vi "HAPS_PhaseSweep_Preamp.vi"() -> ()   [LabVIEW 2023, in "HAPS.lvlib"]
uses:
  HAPS.lvlib
  MCU_Function.ctl
  set_ele.ctl
  HAPS_SerialPort.ctl
  HAPS_MCU_ELE_Func.ctl
  R_S/R_S.lvlib
panel:
  in  "comn_gain":i32=17
  in  "ele_gain":i32=35
  in  "File_note":string
  in  "Init?":bool=TRUE
  out "Duration":dbl
  out "In-Phase : Phase(degree)":dbl[](graph)
  out "In-Phase : Gain(dB)":dbl[](graph)
  out "channel":i32
  out "chain_id":i32
  out "group":i32
  out "array_id":i32
  in  "Phase diff. Criteria":dbl format="%#_13g"
  in  "Tx/Rx":enum16{"Rx", "Tx"}(ring)=enum."Tx"
  in  "array_id (MCU index)":i32
  in  "MCU_UART_addr":refnum<visa-resource-name>="COM8"
  in  "Target(degree)":dbl format="%#_13g"
  in  "SweepPoints":i32=11
  in  "sParameter":i32=21
  in  "Stop_Freq(GHz)":dbl=39.5
  in  "Start_Freq(GHz)":dbl=38.5
  in  "VISA resource name":refnum<visa-resource-name>="TCPIP0::192.168.119.45::inst0::INSTR"
  in  "HAPS_Equipment":enum16{"Keysight", "R&S"}(ring)=enum."R&S"
  # "HAPS_24x24_Phase_Sweep_Preamp"
  # "VNA"
  # "Tx:35\nRx:22"
  # "DUT"
  # "4718.54"
  # "TCPIP0::192.168.1.31::hislip0::INSTR"
  # "Test Status"
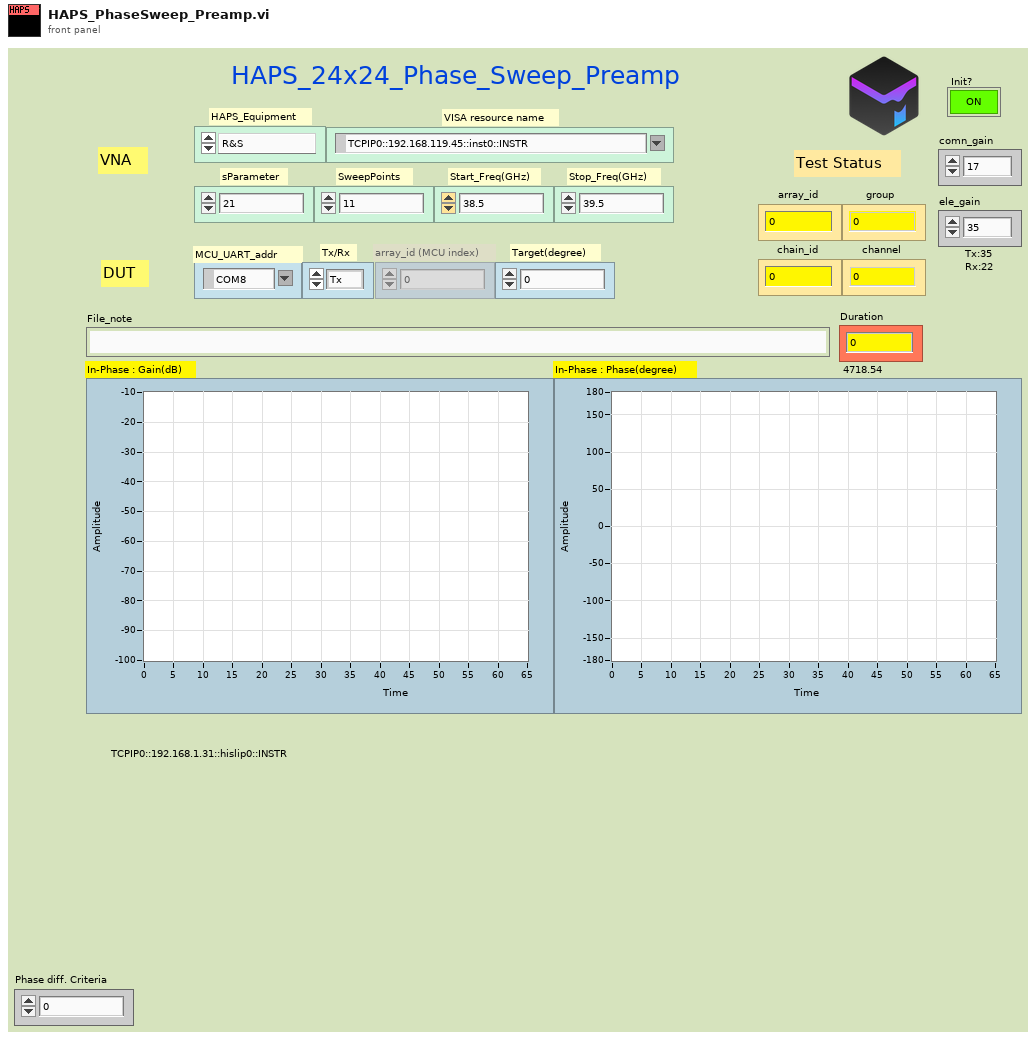
[diagram p1: front panel]
types:
  T1 = typedef "HAPS.lvlib/HAPS_SerialPort.ctl" = enum16{"Init", "Close", "CMD", "Flush"}
  T2 = typedef "HAPS.lvlib/HAPS_MCU_ELE_Func.ctl" = enum16{"array_init", "set_com_gain", "set_ch_gain_phase", "set_pd_range", "get_preamp_temp", "get_bfic_temp", "get_tx_pd", "ch_on", "ch_on_2", "ch_ctrl_all", "array_ctrl_src"}
  T3 = typedef "HAPS.lvlib/MCU_Function.ctl" = cluster{"Tx/Rx":enum16{"Rx", "Tx"}, "Enable?":enum16{"OFF", "On"}, "Source":enum16{"MCU", "ACU"}}
  T4 = typedef "HAPS.lvlib/set_ele.ctl" = cluster{"ch":i32, "chain_id":i32, "group":i32, "array_id":i32, "ele_phase":i32, "ele_gain":i32, "com_gain":i32, "pd_range":i32}
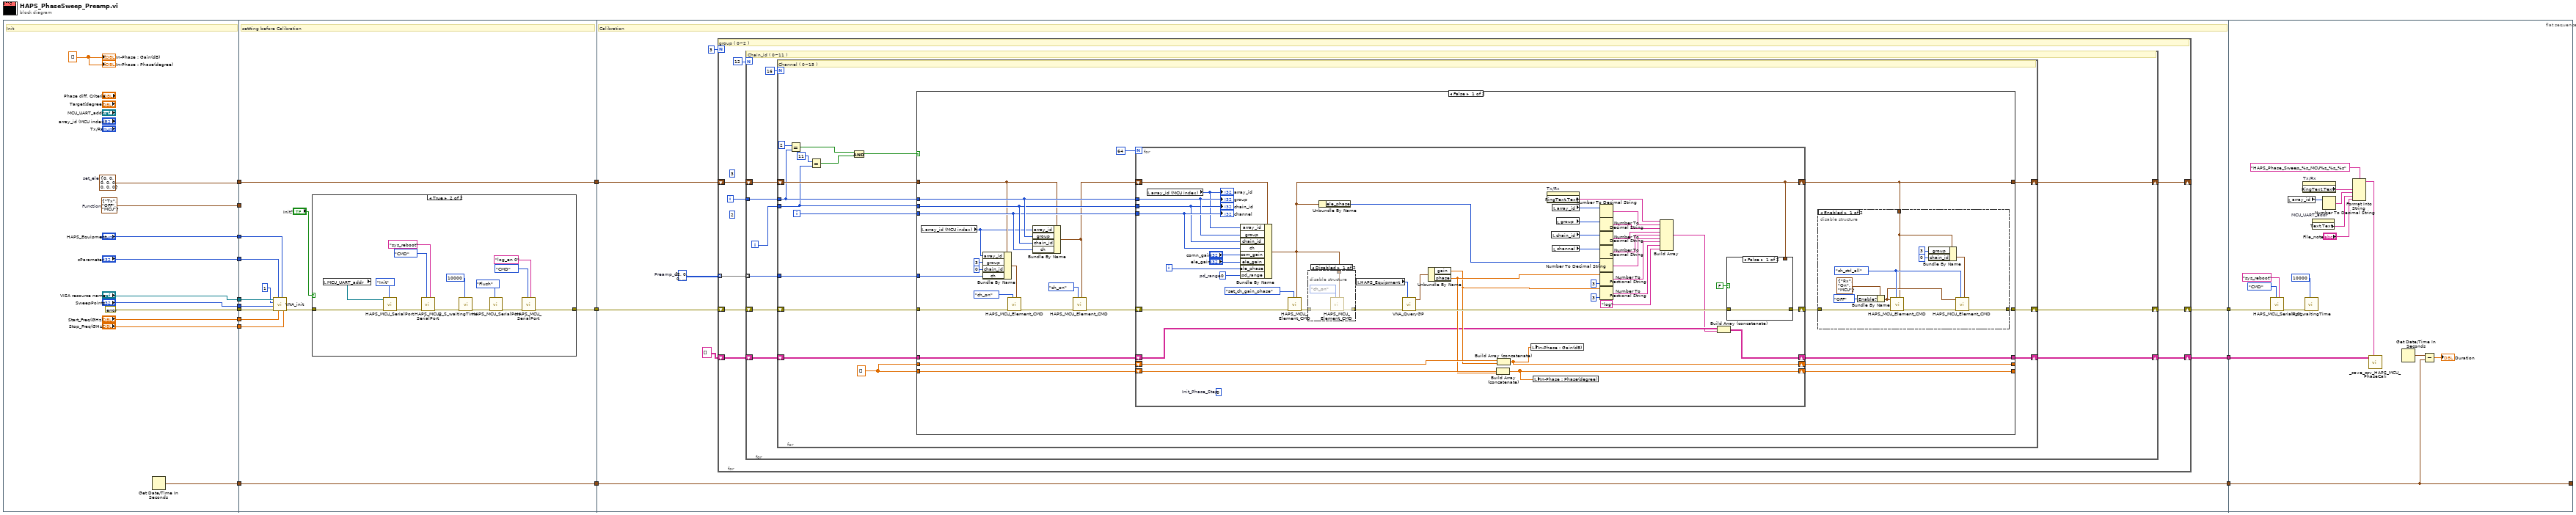
[diagram p0: block diagram]
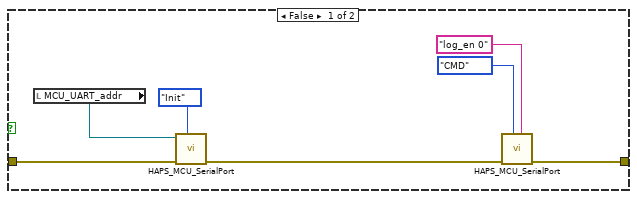
[diagram p2: hidden frame]
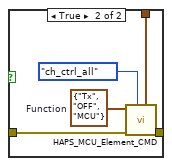
[diagram p5: hidden frame]
diagram:
  n1 = flat-sequence {
    tunnel: [w20] -> w16
    tunnel: [w27] -> w15
    tunnel: [errorcluster {"status"=FALSE, "code"=0, "source"=""} ("error in")] -> w13
    tunnel: ["sParameter"] -> w11
    tunnel: ["VISA resource name"] -> w10
    tunnel: ["Start_Freq(GHz)"] -> w9
    tunnel: ["Stop_Freq(GHz)"] -> w8
    tunnel: ["SweepPoints"] -> w7
    tunnel: ["HAPS_Equipment"] -> w6
    tunnel: [w17] -> w4
    tunnel: w16 -> [w40]
    tunnel: w15 -> [_]
    tunnel: [w40] -> w14
    tunnel: w13 -> [w39]
    tunnel: [w31] -> w12
    tunnel: w11 -> [w38]
    tunnel: w10 -> [w37]
    tunnel: w9 -> [w36]
    tunnel: w8 -> [w35]
    tunnel: w7 -> [w34]
    tunnel: w6 -> [w30]
    tunnel: [w29] -> w5
    tunnel: w4 -> [w29]
    tunnel: w14 -> [w68]
    tunnel: w12 -> [w69]
    tunnel: w5 -> [w65]
    tunnel: [w65] -> w3
    tunnel: [w64] -> w2
    tunnel: [w62] -> w1
    tunnel: [w209] -> _
    tunnel: w3 -> [w209]
    tunnel: w2 -> [w211]
    tunnel: w1 -> [w204]
    frame #0 {
      w18 = dbl[] []
      w20 = T4 {"ch"=0, "chain_id"=0, "group"=0, "array_id"=0, "ele_phase"=0, "ele_gain"=0, "com_gain"=0, "pd_range"=0}  # set_ele
      w27 = T3 {"Tx/Rx"=enum."Tx", "Enable?"=enum."OFF", "Source"=enum."MCU"}  # Function
      # "Init"
      n2 = Get Date/Time In Seconds() -> (seconds since 1Jan1904=w17:timestamp)
      "In-Phase : Gain(dB)" <- w18
      "In-Phase : Phase(degree)" <- w18
    }
    frame #1 {
      # "settting before Calibration"
      n3 = call "VNA_init.vi"("Stop_Freq(GHz)"=w35, "HAPS_MCU_CMD"=w30, "Start_Freq(GHz)"=w36, "sParameter"=w38, "error in"=w39, "SweepPoints"=w34, "Mark no."=1, "VISA resource name"=w37) -> ("error out"=w32:errorcluster)  [unwired: 3 in]
      n4 = case shown="True" "Init?" {
        tunnel: w32 -> [w45 w59]
        tunnel: [w42 w56] -> w31
        frame False {
          n5 = local read "MCU_UART_addr"() -> (w43:refnum<visa-resource-name>)
          n6 = call "HAPS_MCU_SerialPort.vi"("HAPS_SerialPort_Func"=HAPS_SerialPort."Init", "error in"=w45, "VISA resource name"=w43) -> ("error out"=w41:errorcluster)  [unwired: 6 in, 2 out]
          n7 = call "HAPS_MCU_SerialPort.vi"("Command"="log_en 0", "HAPS_SerialPort_Func"=enum16{"Init", "Close", "CMD"}."CMD" ("HAPS_SerialPort"), "error in"=w41) -> ("error out"=w42:errorcluster)  [unwired: 6 in, 2 out]
        }
        frame True {
          n8 = local read "MCU_UART_addr"() -> (w57:refnum<visa-resource-name>)
          n9 = call "HAPS_MCU_SerialPort.vi"("HAPS_SerialPort_Func"=HAPS_SerialPort."Init", "error in"=w59, "VISA resource name"=w57) -> ("error out"=w53:errorcluster)  [unwired: 6 in, 2 out]
          n10 = call "HAPS_MCU_SerialPort.vi"("Command"="sys_reboot", "HAPS_SerialPort_Func"=enum16{"Init", "Close", "CMD"}."CMD" ("HAPS_SerialPort"), "error in"=w53) -> ("error out"=w52:errorcluster)  [unwired: 6 in, 2 out]
          n11 = call "R_S_waitingTime.vi"("Waiting Time(ms)"=u32 10000, "error in"=w52) -> ("error out"=w50:errorcluster)  [unwired: 9 in]
          n12 = call "HAPS_MCU_SerialPort.vi"("HAPS_SerialPort_Func"=HAPS_SerialPort."Flush", "error in"=w50) -> ("error out"=w48:errorcluster)  [unwired: 7 in, 2 out]
          n13 = call "HAPS_MCU_SerialPort.vi"("Command"="log_en 0", "HAPS_SerialPort_Func"=enum16{"Init", "Close", "CMD"}."CMD" ("HAPS_SerialPort"), "error in"=w48) -> ("error out"=w56:errorcluster)  [unwired: 6 in, 2 out]
        }
      }
    }
    frame #2 {
      w63 = i32[][] [[2, 0, 0, 8, 8, 10, 11, 9, 9, 1, 1, 3], [3, 1, 1, 9, 9, 11, 13, 15, 15, 7, 7, 5], [5, 7, 7, 15, 15, 13, 14, 14, 6, 6, 4, 12]]  # Preamp_ch
      # "Calibration"
      n14 = for {
        N: 3 -> [_]
        shift-right: [w78] -> _
        shift-left: w68 -> [w74]
        shift-right: [w77] -> w64
        shift-left: string[][] [] -> [w73]
        shift-right: [w76] -> w62
        shift-left: w69 -> [w75]
        tunnel: w63 -> [w70] mode=indexing
        i -> [w71]
        (unwired) 2
        (unwired) 3
        # "group ( 0~2 )"
        n15 = for {
          N: 12 -> [_]
          shift-right: [w87] -> w78
          shift-left: w74 -> [w84]
          shift-right: [w86] -> w77
          shift-left: w73 -> [w83]
          shift-right: [w80] -> w76
          shift-left: w75 -> [w85]
          tunnel: w71 -> [w82]
          tunnel: w70 -> [w79] mode=indexing
          i -> [w81]
          # "Chain_id ( 0~11 )"
          n16 = for {
            N: 16 -> [_]
            shift-right: [w101] -> w87
            shift-left: w84 -> [w104]
            shift-right: [w99] -> w86
            shift-left: w83 -> [w100]
            shift-right: [w102] -> w80
            shift-left: w85 -> [w103]
            tunnel: w82 -> [w98]
            tunnel: w81 -> [w90]
            tunnel: w79 -> [w89]
            i -> [w91]
            w92 = dbl[] []
            # "Channel ( 0~15 )"
            n17 = Equal?(x=2, y=w98) -> (x = y?=w95:bool)
            n18 = Equal?(x=11, y=w90) -> (x = y?=w94:bool)
            n19 = And(x=w95, y=w94) -> (x .and. y?=w93:bool)
            n20 = case shown="False" w93 {
              tunnel: w104 -> [w111 w198]
              tunnel: w91 -> [w120 _]
              tunnel: w103 -> [w112 w197]
              tunnel: w98 -> [w122 _]
              tunnel: w90 -> [w121 _]
              tunnel: w92 -> [w129 w200]
              tunnel: w92 -> [w128 w201]
              tunnel: [w127 w200] -> _
              tunnel: [w126 w201] -> _
              tunnel: [w116 w197] -> w102
              tunnel: [w115 w198] -> w101
              tunnel: w100 -> [w124 w199]
              tunnel: [w123 w199] -> w99
              tunnel: w89 -> [w105 _]
              frame False {
                n21 = local read "array_id (MCU index)"() -> (w109:i32)
                n22 = Bundle By Name(cluster=w111, "array_id"=w109, "group"=3, "chain_id"=0, "ch"=w105) -> (w110:T4)
                n23 = call "HAPS_MCU_Element_CMD.vi"("set_ele"=w110, "HAPS_MCU_ELE_Func."=HAPS_MCU_ELE_Func."ch_on", "error in"=w112) -> ("error out"=w113:errorcluster)  [unwired: 7 in, 1 out]
                n24 = Bundle By Name(cluster=w111, "array_id"=w109, "group"=w122, "chain_id"=w121, "ch"=w120) -> (w106:T4)
                n25 = call "HAPS_MCU_Element_CMD.vi"("set_ele"=w106, "HAPS_MCU_ELE_Func."=HAPS_MCU_ELE_Func."ch_on", "error in"=w113) -> ("error out"=w118:errorcluster)  [unwired: 7 in, 1 out]
                n26 = for {
                  N: 64 -> [_]
                  tunnel: w120 -> [w184]
                  tunnel: w122 -> [w182]
                  tunnel: w121 -> [w181]
                  shift-right: [w157] -> w127
                  shift-left: w129 -> [w159]
                  shift-right: [w156] -> w126
                  shift-left: w128 -> [w158]
                  shift-right: [w153] -> w117
                  shift-left: w118 -> [w183]
                  shift-right: [w143] -> w115
                  shift-left: w106 -> [w185]
                  shift-right: [w147] -> w123
                  shift-left: w124 -> [w149]
                  i -> [w155]
                  w179 = 0  # pd_range
                  (unwired) 0  # Init_Phase_Step
                  n27 = local read "array_id (MCU index)"() -> (w177:i32)
                  "array_id" <- w177
                  n28 = Bundle By Name(cluster=w185, "array_id"=w177, "group"=w182, "chain_id"=w181, "ch"=w184, "com_gain"="comn_gain", "ele_gain"="ele_gain", "ele_phase"=w155, "pd_range"=w179) -> (w143:T4)
                  n29 = call "HAPS_MCU_Element_CMD.vi"("set_ele"=w143, "HAPS_MCU_ELE_Func."=HAPS_MCU_ELE_Func."set_ch_gain_phase", "error in"=w183) -> ("error out"=w145:errorcluster)  [unwired: 7 in, 1 out]
                  n30 = disable-structure shown="Disabled" {
                    disable-tunnel: w145 -> [w189 w190]
                    disable-tunnel: [w188 w190] -> w144
                    disable-tunnel: w143 -> [w186 _]
                    frame Disabled {
                      n31 = call "HAPS_MCU_Element_CMD.vi"("set_ele"=w186, "HAPS_MCU_ELE_Func."=HAPS_MCU_ELE_Func."ch_on", "error in"=w189) -> ("error out"=w188:errorcluster)  [unwired: 7 in, 1 out]
                    }
                    frame Enabled {
                    }
                  }
                  n32 = Unbundle By Name(w143) -> ("ele_phase"=w152:i32)
                  n33 = local read "HAPS_Equipment"() -> (w161:enum16{"Keysight", "R&S"})
                  n34 = call "VNA_QueryGP.vi"("HAPS_Equipment"=w161, "error in"=w144) -> ("error out"=w154:errorcluster, "queryMarker"=w160:cluster{"gain":dbl, "phase":dbl})  [unwired: 8 in]
                  n35 = Unbundle By Name(w160) -> ("gain"=w150:dbl, "phase"=w151:dbl)
                  n36 = Build Array (concatenate)(w158, w151) -> (w156:dbl[])
                  n37 = Build Array (concatenate)(w159, w150) -> (w157:dbl[])
                  n38 = local write "In-Phase : Gain(dB)"(w157) -> ()
                  n39 = local write "In-Phase : Phase(degree)"(w156) -> ()
                  n40 = property on="Tx/Rx" class="Enum (strict)"() -> ("RingText.Text"=w166:string)  [unwired: 2 in, 2 out]
                  n41 = local read "chain_id"() -> (w163:i32)
                  n42 = local read "array_id"() -> (w165:i32)
                  n43 = local read "channel"() -> (w162:i32)
                  n44 = local read "group"() -> (w164:i32)
                  n45 = Number To Decimal String(number=w165) -> (decimal integer string=w167:string)  [unwired: 1 in]
                  n46 = Number To Decimal String(number=w164) -> (decimal integer string=w168:string)  [unwired: 1 in]
                  n47 = Number To Decimal String(number=w163) -> (decimal integer string=w169:string)  [unwired: 1 in]
                  n48 = Number To Decimal String(number=w162) -> (decimal integer string=w170:string)  [unwired: 1 in]
                  n49 = Number To Decimal String(number=w152) -> (decimal integer string=w171:string)  [unwired: 1 in]
                  n50 = Number To Fractional String(number=w151, precision (6)=i16 3) -> (F-format string=w174:string)  [unwired: 2 in]
                  n51 = Number To Fractional String(number=w150, precision (6)=i16 3) -> (F-format string=w175:string)  [unwired: 2 in]
                  n52 = Build Array(w166, w167, w168, w169, w170, w171, w174, w175, "log") -> (w148:string[])
                  n53 = Build Array (concatenate)(w149, w148) -> (w147:string[][])
                  n54 = case shown="False" FALSE {
                    tunnel: w154 -> [w191 w194]
                    tunnel: [w191 w193] -> w153
                    tunnel: w143 -> [_ w192]
                    frame False {
                    }
                    frame True {
                      w196 = T3 {"Tx/Rx"=enum."Tx", "Enable?"=enum."OFF", "Source"=enum."MCU"}  # Function
                      n55 = call "HAPS_MCU_Element_CMD.vi"("set_ele"=w192, "HAPS_MCU_ELE_Func."=HAPS_MCU_ELE_Func."ch_ctrl_all", "error in"=w194, "Function"=w196) -> ("error out"=w193:errorcluster)  [unwired: 6 in, 1 out]
                    }
                  }
                  "group" <- w182
                  "chain_id" <- w181
                  "channel" <- w184
                }
                n56 = disable-structure shown="Enabled" {
                  disable-tunnel: w117 -> [w140 w141]
                  disable-tunnel: [w136 w141] -> w116
                  disable-tunnel: w115 -> [w130 _]
                  frame Enabled {
                    w135 = HAPS_MCU_ELE_Func."ch_ctrl_all" ("HAPS_MCU_ELE_Func.")
                    n57 = Bundle By Name(cluster=T3 {"Tx/Rx"=enum."Rx", "Enable?"=enum."On", "Source"=enum."MCU"} ("Function"), "Enable?"=enum16{"OFF", "On"}."OFF") -> (w134:T3)
                    n58 = call "HAPS_MCU_Element_CMD.vi"("set_ele"=w130, "HAPS_MCU_ELE_Func."=w135, "error in"=w140, "Function"=w134) -> ("error out"=w137:errorcluster)  [unwired: 6 in, 1 out]
                    n59 = Bundle By Name(cluster=w130, "group"=3, "chain_id"=0) -> (w131:T4)
                    n60 = call "HAPS_MCU_Element_CMD.vi"("set_ele"=w131, "HAPS_MCU_ELE_Func."=w135, "error in"=w137, "Function"=w134) -> ("error out"=w136:errorcluster)  [unwired: 6 in, 1 out]
                  }
                  frame Disabled {
                  }
                }
              }
              frame True {
              }
            }
          }
        }
      }
    }
    frame #3 {
      n61 = call "HAPS_MCU_SerialPort.vi"("Command"="sys_reboot", "HAPS_SerialPort_Func"=enum16{"Init", "Close", "CMD"}."CMD" ("HAPS_SerialPort"), "error in"=w204) -> ("error out"=w202:errorcluster)  [unwired: 6 in, 2 out]
      n62 = local read "array_id"() -> (w214:i32)
      n63 = property on="Tx/Rx" class="Enum (strict)"() -> ("RingText.Text"=w213:string)  [unwired: 2 in, 2 out]
      n64 = call "R_S_waitingTime.vi"("Waiting Time(ms)"=u32 10000, "error in"=w202) -> ()  [unwired: 9 in, 1 out]
      n65 = property on="MCU_UART_addr" class="VISAName"() -> ("Text.Text"=w217:string)  [unwired: 2 in, 2 out]
      n66 = Number To Decimal String(number=w214) -> (decimal integer string=w215:string)  [unwired: 1 in]
      n67 = Format Into String(format string="HAPS_Phase_Sweep_%s_MCU%s_%s_%s", w213, w215, w217, "File_note") -> (resulting string=w216:string)  [unwired: 2 in, 1 out]
      n68 = call "_save_csv_HAPS_MCU_PhaseCali.vi"("NoteName"=w216, "array in"=w211) -> ()  [unwired: 9 in, 1 out]
      n69 = Get Date/Time In Seconds() -> (seconds since 1Jan1904=w210:timestamp)
      n70 = Subtract(x=w210, y=w209) -> (x-y=→"Duration":dbl)
    }
  }
